vi "cmd move.vi"(8 "error in (no error)":errorcluster, 9 "new Value":variant, 11 "motor in":refnum<class "AISAS motor.lvclass">) -> (0 "error out":errorcluster, 1 "Response":u8 format="%x", 3 "motor out":refnum<class "AISAS motor.lvclass">, 5 "Motor Ok?":bool, 7 "Log response":string)   [LabVIEW 2014, in "AISAS motor.lvclass"]
uses:
  AISAS motor.lvclass
  Controls/motor.ctl
  AISAS motor.lvclass/AISAS motor.ctl
panel:
  out "Motor":T1
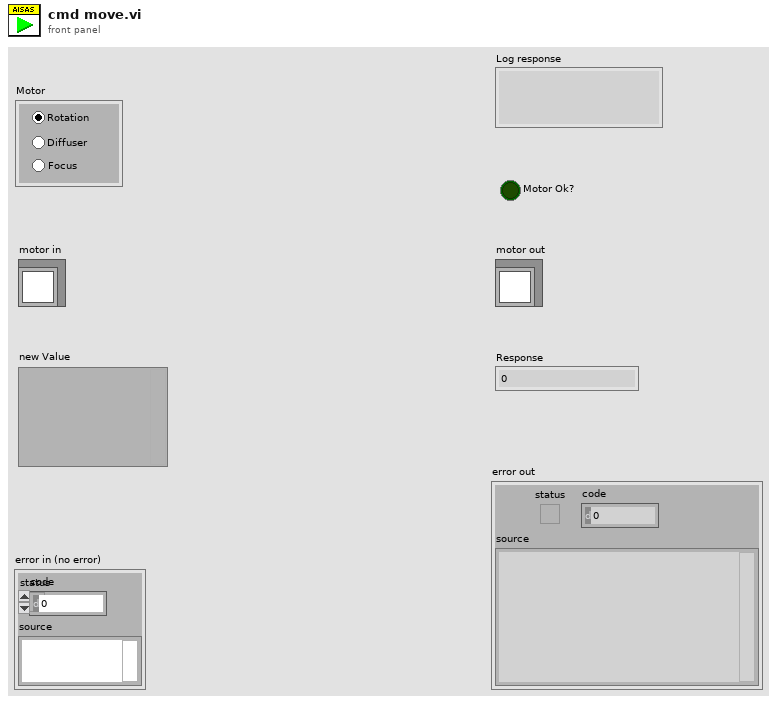
[diagram p1: front panel]
types:
  T1 = typedef "motor.ctl" = enum32{"Rotation", "Diffuser ", "Focus"}
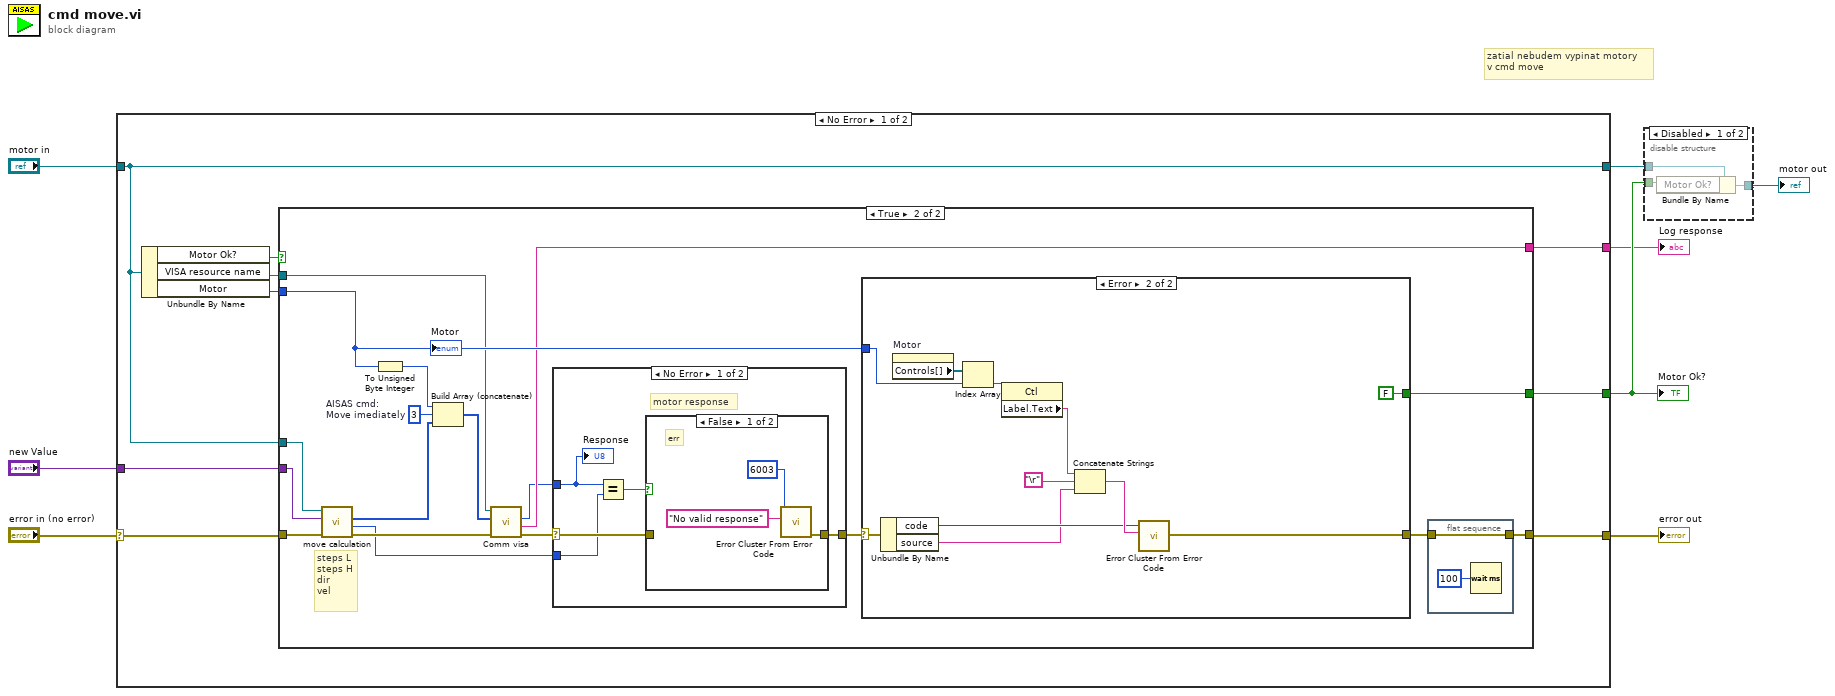
[diagram p0: block diagram]
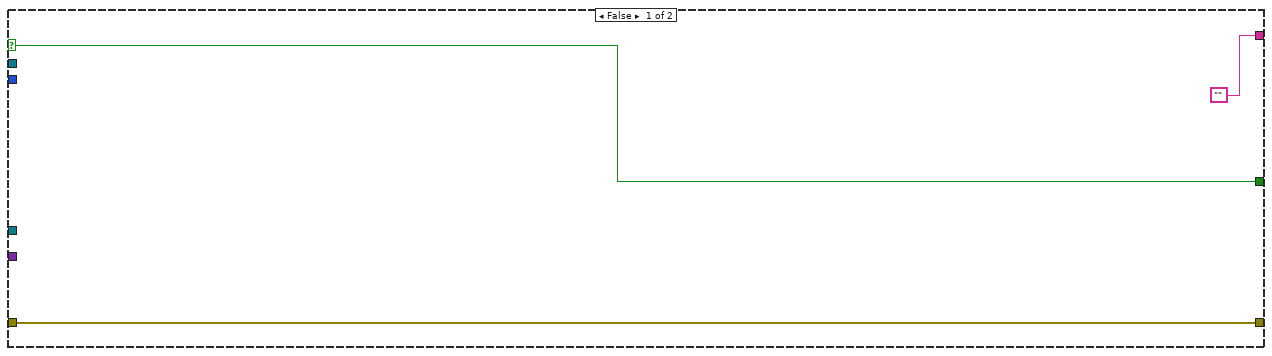
[diagram p3: hidden frame]
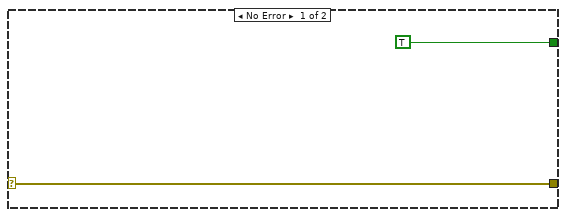
[diagram p4: hidden frame]
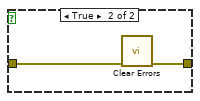
[diagram p5: hidden frame]
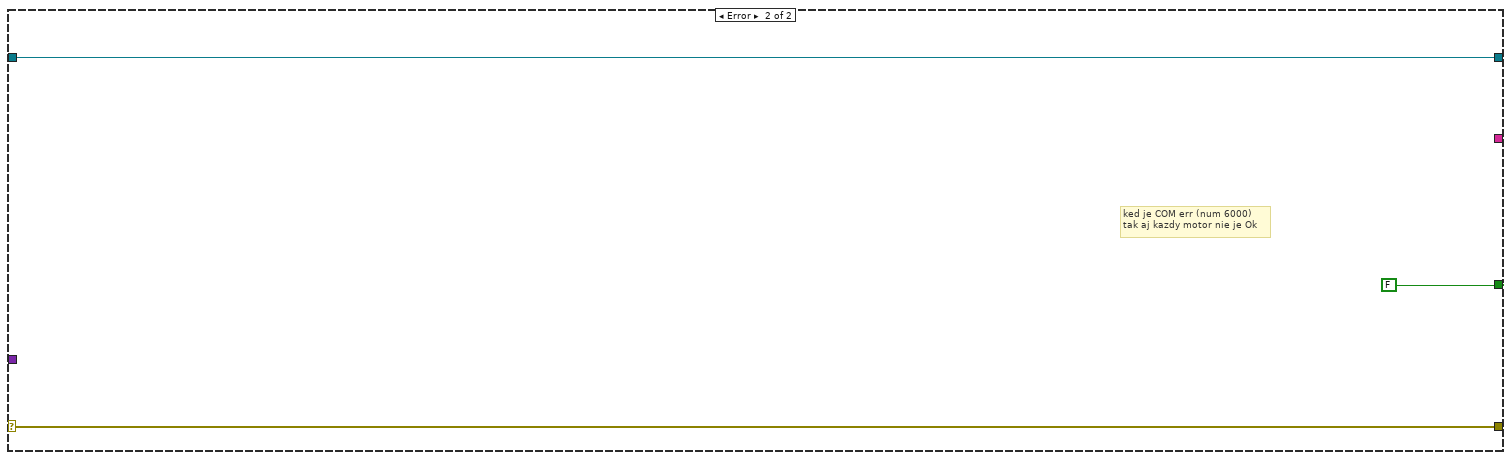
[diagram p7: hidden frame]
diagram:
  # "zatial nebudem vypinat motory\nv cmd move"
  n1 = case shown="No Error" "error in (no error)" {
    selector: "error in (no error)" -> [w15 w67]
    tunnel: [w17 w67] -> w7
    tunnel: "motor in" -> [w13 w66]
    tunnel: [w14 FALSE ("Motor Ok")] -> w5
    tunnel: [w13 w66] -> w4
    tunnel: "new Value" -> [w12 _]
    tunnel: [w9 _] -> w1
    frame No Error {
      n2 = Unbundle By Name(w13) -> ("Motor Ok?"=w10:bool, "VISA resource name"=w11:refnum<visa-resource-name>, "Motor"=w16:T1)
      n3 = case shown="True" w10 {
        selector: w10 -> [w18 _]
        tunnel: [w18 w37] -> w14
        tunnel: [w20 w30] -> w17
        tunnel: w16 -> [_ w35]
        tunnel: w11 -> [_ w21]
        tunnel: w15 -> [w20 w27]
        tunnel: ["" w32] -> w9
        tunnel: w13 -> [_ w24]
        tunnel: w12 -> [_ w23]
        frame False {
        }
        frame True {
          w28 = u8 3  # AISAS cmd: Move imediately
          # "steps L\nsteps H\ndir\nvel"
          n4 = call "move calculation.vi"("error in (no error)"=w27, "new Value"=w23, "AISAS motor in"=w24) -> ("error out"=w26:errorcluster, "Motor Direction"=w22:u8, "Move param"=w25:u8[])  [unwired: 5 in, 1 out]
          n5 = To Unsigned Byte Integer(number=w35) -> (unsigned 8bit integer=w34:u8)
          n6 = Build Array (concatenate)(w34, w28, w25) -> (w33:u8[])
          n7 = call "Comm visa.vi"("error in (no error)"=w26, "Command"=w33, "VISA in"=w21) -> ("error out"=w36:errorcluster, "status log"=w32:string, "Response"=w29:u8)  [unwired: 5 in, 1 out]
          n8 = case shown="No Error" w36 {
            selector: w36 -> [w58 w64]
            tunnel: [w57 w64] -> w38
            tunnel: w29 -> [w56 _]
            tunnel: w22 -> [w55 _]
            frame No Error {
              # "motor response"
              n9 = Equal?(x=w56, y=w55) -> (x = y?=w54:bool)
              n10 = case shown="False" w54 {
                tunnel: w58 -> [_ w63]
                tunnel: [w59 w62] -> w57
                frame False {
                  # "err"
                  n11 = call <vilib>:"Error Cluster From Error Code.vi"("error message (\"\")"="No valid response" ("error message (\"\")"), "error code (0)"=6003) -> ("error out"=w59:errorcluster)  [unwired: 7 in]
                }
                frame True {
                  n12 = call <vilib>:"Clear Errors.vi"("error in (no error)"=w63) -> ("error out"=w62:errorcluster)  [unwired: 5 in, 1 out]
                }
              }
              "Response" <- w56
            }
            frame Error {
            }
          }
          n13 = case shown="Error" w38 {
            selector: w38 -> [w41 w49]
            tunnel: [TRUE ("Motor Ok") FALSE ("Motor Ok")] -> w37
            tunnel: w35 -> [_ w50]
            tunnel: [w41 w43] -> w31
            frame No Error {
            }
            frame Error {
              n14 = Unbundle By Name(w49) -> ("code"=w47:i32, "source"=w46:string)
              n15 = property on="Motor" class="RadioBtnsControl (strict)"() -> ("Controls[]"=w52:refnum<vi>[])  [unwired: 2 in, 2 out]
              n16 = Index Array(array=w52, index=w50) -> (element=w51:refnum<vi>)
              n17 = property class="Ctl"(reference=w51) -> ("Label.Text"=w45:string)  [unwired: 1 in, 2 out]
              n18 = Concatenate Strings(w45, "\r", w46) -> (w48:string)
              n19 = call <vilib>:"Error Cluster From Error Code.vi"("error message (\"\")"=w48, "error code (0)"=w47) -> ("error out"=w43:errorcluster)  [unwired: 7 in]
            }
          }
          n20 = flat-sequence {
            tunnel: w31 -> [w40]
            tunnel: [w40] -> w30
            frame #0 {
              n21 = Wait (ms)(milliseconds to wait=u32 100) -> ()  [unwired: 1 out]
            }
          }
          "Motor" <- w35
        }
      }
    }
    frame Error {
      # "ked je COM err (num 6000)\ntak aj kazdy motor nie je Ok"
    }
  }
  "error out" <- w7
  "Motor Ok?" <- w5
  "Log response" <- w1
  n22 = disable-structure shown="Disabled" {
    disable-tunnel: w5 -> [w70 _]
    disable-tunnel: w4 -> [w69 w71]
    disable-tunnel: [w68 w71] -> w3
    frame Disabled {
      n23 = Bundle By Name(cluster=w69, "Motor Ok?"=w70) -> (w68:refnum<class "AISAS motor.lvclass">)
    }
    frame Enabled {
    }
  }
  "motor out" <- w3
